vi "Write RetentionPolicy.vi"(10 "RetentionPolicy.lvclass":refnum<class "RetentionPolicy.lvclass">, 11 "DataPoint in":refnum<class "DataPoint.lvclass">) -> (3 "DataPoint out":refnum<class "DataPoint.lvclass">)   [LabVIEW 2018, in "InfluxDB Client.lvlib" / "DataPoint.lvclass"]
uses:
  DataPoint.lvclass
  RetentionPolicy/RetentionPolicy.lvclass
  DataPoint.lvclass/DataPoint.ctl
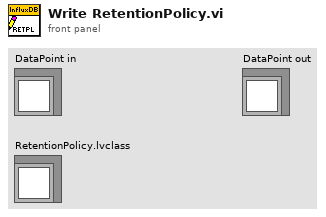
[diagram p1: front panel]
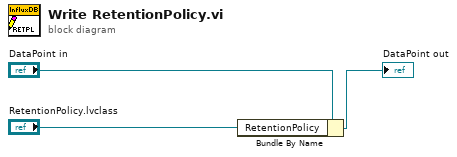
[diagram p0: block diagram]
diagram:
  n1 = Bundle By Name(cluster="DataPoint in", "RetentionPolicy"="RetentionPolicy.lvclass") -> (→"DataPoint out":refnum<class "DataPoint.lvclass">)
